vi "Read State.vi"(8 "error in (no error)":errorcluster, 10 "Trigger":bool, 11 "ExtFlatShutt in":refnum<class "ExtFlatShutt.lvclass">) -> (0 "error out":errorcluster, 2 "Set":T1, 3 "ExtFlatShutt out":refnum<class "ExtFlatShutt.lvclass">)   [LabVIEW 2016, in "ExtFlatShutt.lvclass"]
uses:
  ExtFlatShutt.lvclass
  Controls/Shutter States.ctl
  Shutter.lvclass
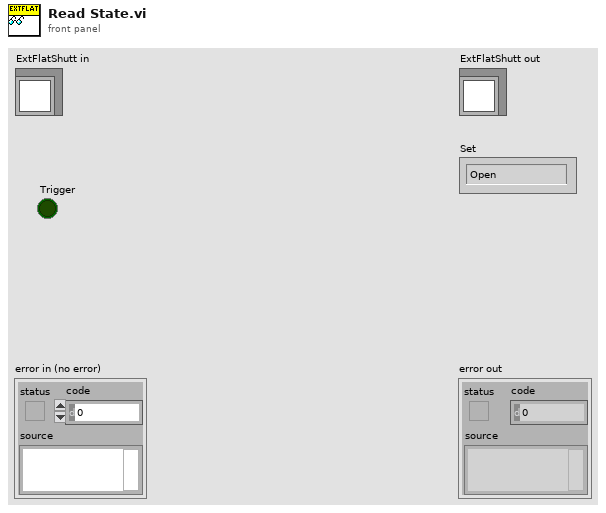
[diagram p1: front panel]
types:
  T1 = typedef "Shutter States.ctl" = enum16{"Open", "Close", "Wait", "Off", "Arm", "Idle"}
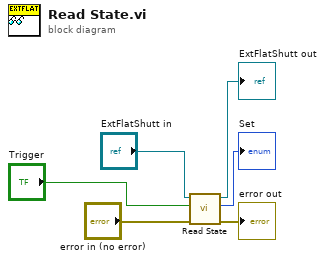
[diagram p0: block diagram]
diagram:
  n1 = call-parent "Read State.vi"("error in (no error)"="error in (no error)", "Trigger"="Trigger", "Shutter in"="ExtFlatShutt in") -> ("error out"=→"error out":errorcluster, "Set"=→"Set":T1, "Shutter out"=→"ExtFlatShutt out":refnum<class "ExtFlatShutt.lvclass">)  [unwired: 6 in]
